vi "Check_Timer.vi"(8 "error in (no error)":errorcluster, 11 "Logger_Data In":T1) -> (0 "error out":errorcluster, 2 "Time has Elapsed":bool, 3 "Logger_Data Out":T1)   [LabVIEW 2019, in "Data_Logger.lvlib"]
uses:
  Data_Logger.lvlib
  Logger_Data.ctl
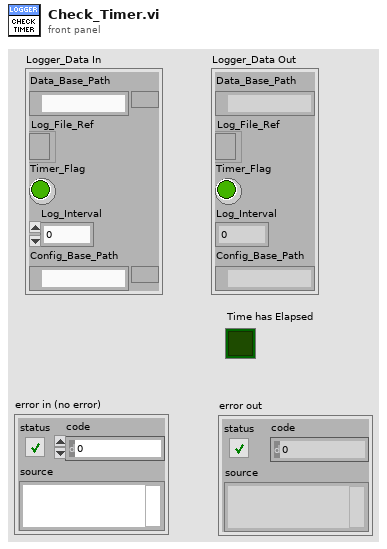
[diagram p1: front panel]
types:
  T1 = typedef "Data_Logger.lvlib/Logger_Data.ctl" = cluster{"Data_Base_Path":path, "Log_File_Ref":refnum<file>, "Timer_Flag":bool, "Log_Interval":dbl, "Config_Base_Path":path}
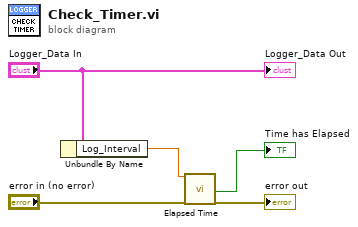
[diagram p0: block diagram]
diagram:
  n1 = Unbundle By Name("Logger_Data In") -> ("Log_Interval"=w3:dbl)
  n2 = call "Elapsed Time"("Time Target (s)"=w3, "error in (no error)"="error in (no error)") -> ("Time has Elapsed"=→"Time has Elapsed":bool, "error out"=→"error out":errorcluster)  [unwired: 10 in, 6 out]
  "Logger_Data Out" <- "Logger_Data In"
